vi "st_eval CDF (bin kx).vi"(4 "parameters":variant, 5 "x":dbl) -> (2 "f(x)":dbl)   [LabVIEW 2010, in "NI_Gmath.lvlib"]
uses:
  NI_Gmath.lvlib
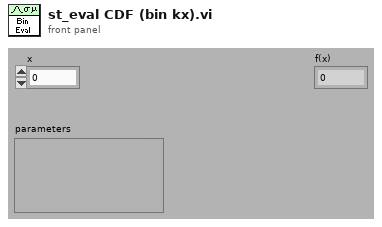
[diagram p1: front panel]
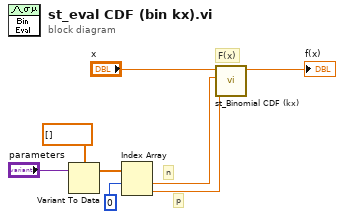
[diagram p0: block diagram]
diagram:
  # "p"
  # "n"
  # "F(x)"
  n1 = Variant To Data(Variant="parameters", type=dbl[] []) -> (data=w6:dbl[])  [unwired: 1 in, 1 out]
  n2 = Index Array(array=w6, index #1=0 ("index")) -> (element #1=w4:dbl, element #2=w3:dbl)  [unwired: 1 in]
  n3 = call "st_Binomial CDF (kx).vi"("a"=w3, "n"=w4, "x"="x") -> ("cdf(x)"=→"f(x)":dbl)  [unwired: 7 in, 1 out]
